vi "Evaluate Part 2.vi"() -> ()   [LabVIEW 2020]
uses:
  Galaxy/Galaxy.lvclass
panel:
  out "sum":u64
  in  "Input":string="...#......\n.......#..\n#.........\n..........\n......#...\n.#........\n.........#\n..........\n.......#..\n#...#....."
  # "618719584 too low"
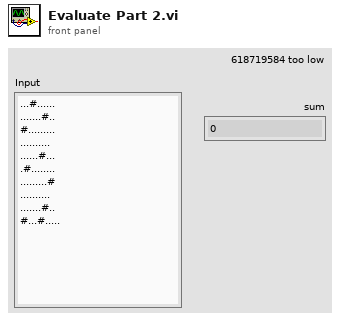
[diagram p1: front panel]
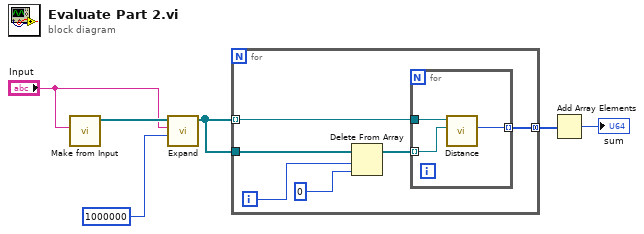
[diagram p0: block diagram]
diagram:
  n1 = call "Make from Input.vi"("Input"="Input") -> ("Galaxy out"=w6:refnum<class "Galaxy.lvclass">[])  [unwired: 9 in, 1 out]
  n2 = call "Expand.vi"("Factor"=1000000, "Input"="Input", "Galaxy in"=w6) -> ("Array"=w4:refnum<class "Galaxy.lvclass">[])  [unwired: 7 in, 1 out]
  n3 = for {
    tunnel: w4 -> [w12] mode=indexing
    tunnel: w4 -> [w11]
    tunnel: [w7] -> w3 mode=concatenating
    i -> [w10]
    n4 = Delete From Array(array=w11, length=w10, index=0) -> (array with subset deleted=w8:refnum<class "Galaxy.lvclass">[])  [unwired: 1 out]
    n5 = for {
      tunnel: w12 -> [w15]
      tunnel: w8 -> [w14] mode=indexing
      tunnel: [w13] -> w7 mode=indexing
      n6 = call "Distance.vi"("Galaxy in 2"=w14, "Galaxy in"=w15) -> ("Numeric"=w13:u64)  [unwired: 8 in, 1 out]
    }
  }
  n7 = Add Array Elements(numeric array=w3) -> (sum=→"sum":u64)
